vi "Set View by Listbox Index.vi"(8 "error in (no error)":errorcluster, 10 "Index":i32, 11 "LeftListboxViewManager In":refnum<class "LeftListboxViewManager.lvclass">) -> (0 "error out":errorcluster, 3 "LeftListboxViewManager Out":refnum<class "LeftListboxViewManager.lvclass">)   [LabVIEW 2020, in "MVA Framework.lvlib" / "LeftListboxViewManager.lvlib" / "LeftListboxViewManager.lvclass"]
doc: "按列表框索引设置视图"
uses:
  LeftListboxViewManager.lvclass
  modules/mva-viewable/Source/IViewManager/IViewManager/IViewManager.lvclass/IViewManager.ctl
  LeftListboxViewManager.lvclass/LeftListboxViewManager.ctl
  modules/mva-viewable/Source/IViewable/IViewable Messages/Insert Front Panel Msg/Insert Front Panel Msg.lvclass/Insert Front Panel Msg.ctl
  <vilib>/ActorFramework/Message Enqueuer/Message Enqueuer.lvclass/Message Enqueuer.ctl
  <vilib>/ActorFramework/Message Enqueuer/Enqueue.vi
  modules/mva-viewable/Source/IViewable/IViewable Messages/Insert Front Panel Msg/Insert Front Panel Msg.lvclass
  C:/Program Files/National Instruments/LabVIEW 2020/vi.lib/ActorFramework/Message/Message.lvclass
  <vilib>/ActorFramework/Message Priority Queue/Priority Enqueue.vi
  modules/mva-viewable/Source/IViewManager/IViewManager/IViewManager.lvclass
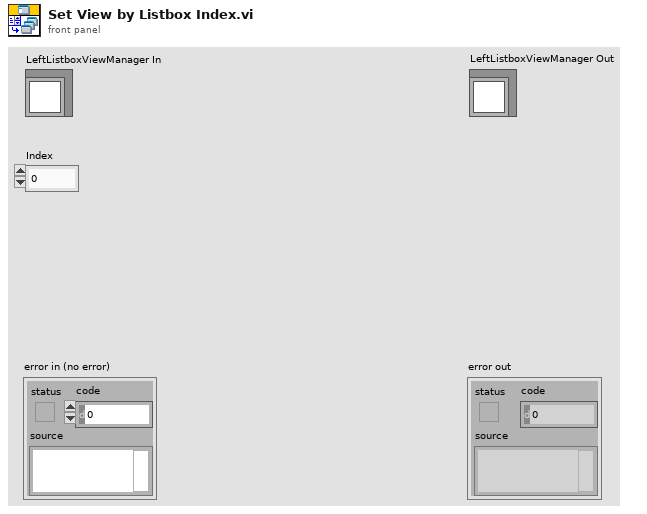
[diagram p1: front panel]
types:
  T1 = typedef "MVA Framework.lvlib/IViewable.lvlib/ProtectedSubpanel.lvclass/Protected Subpanel Reference.ctl" = refnum<data-value>
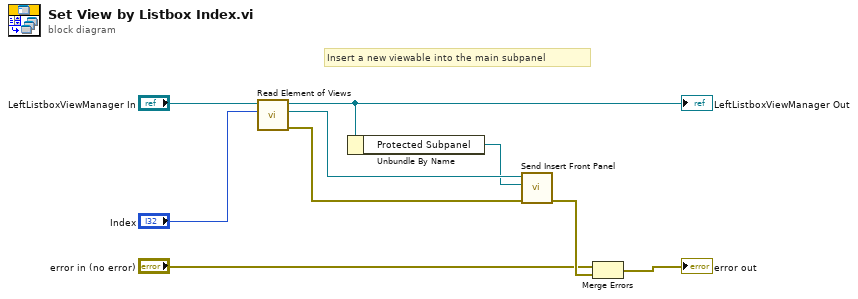
[diagram p0: block diagram]
diagram:
  # "Insert a new viewable into the main subpanel"
  n1 = call "Read Element of Views.vi"("Index"="Index", "IViewManager In"="LeftListboxViewManager In") -> ("error out"=w5:errorcluster, "View Ref"=w6:refnum<class "Message Enqueuer.lvclass">, "IViewManager Out"=w7:refnum<class "LeftListboxViewManager.lvclass">)  [unwired: 7 in]
  "LeftListboxViewManager Out" <- w7
  n2 = Unbundle By Name(w7) -> ("Protected Subpanel"=w4:T1)
  n3 = call "Send Insert Front Panel.vi"("error in (no error)"=w5, "Protected Subpanel"=w4, "Message Enqueuer"=w6) -> ("error out"=w9:errorcluster)  [unwired: 7 in, 1 out]
  n4 = Merge Errors("error in (no error)", w9) -> (→"error out":errorcluster)
